vi "Add Noise.vi"(6 "Sampling":T1 {"Fs" format="%#_13g"}, 8 "error in (no error)":errorcluster, 11 "AI []":waveform(dbl)[](array[waveform])) -> (0 "error out":errorcluster, 3 "AI + Noise":waveform(dbl)[](array[waveform]))   [LabVIEW 2019, in "Instrument.Lockin.lvlib" / "Instrument.DAQ.lvclass"]
uses:
  Instrument.DAQ.lvclass
  Typedefs/DAQ.Sampling.Sampling--Cluster.ctl
  <vilib>/measure/maspectr.llb/FFT Power Spectrum and PSD for N Chan.vi
  <vilib>/measure/NI_MABase.lvlib
  <vilib>/measure/NI_MAPro.lvlib
panel:
  out "Waveform Graph":cluster{"f0":dbl, "df":dbl, "magnitude":dbl[]}[](graph)
  in  "Noise Cluster":T2={"1/f vs. Uniform "=1.0, "60Hz Amplitude"=0.005, "Gauss/Unif %"=0.5, "Noise Amp"=0.005}
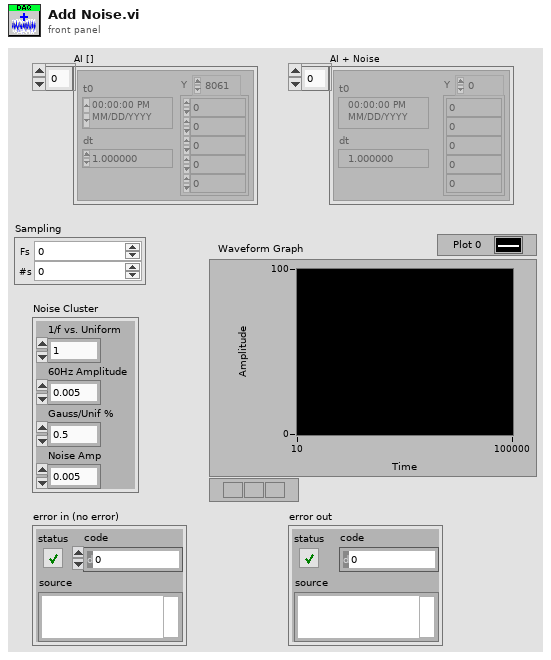
[diagram p1: front panel]
types:
  T1 = typedef "Instrument.Lockin.lvlib/Instrument.DAQ.lvclass/DAQ.Sampling.Sampling--Cluster.ctl" = cluster{"Fs":dbl, "#s":i32}
  T2 = cluster{"1/f vs. Uniform ":dbl, "60Hz Amplitude":dbl, "Gauss/Unif %":dbl, "Noise Amp":dbl}
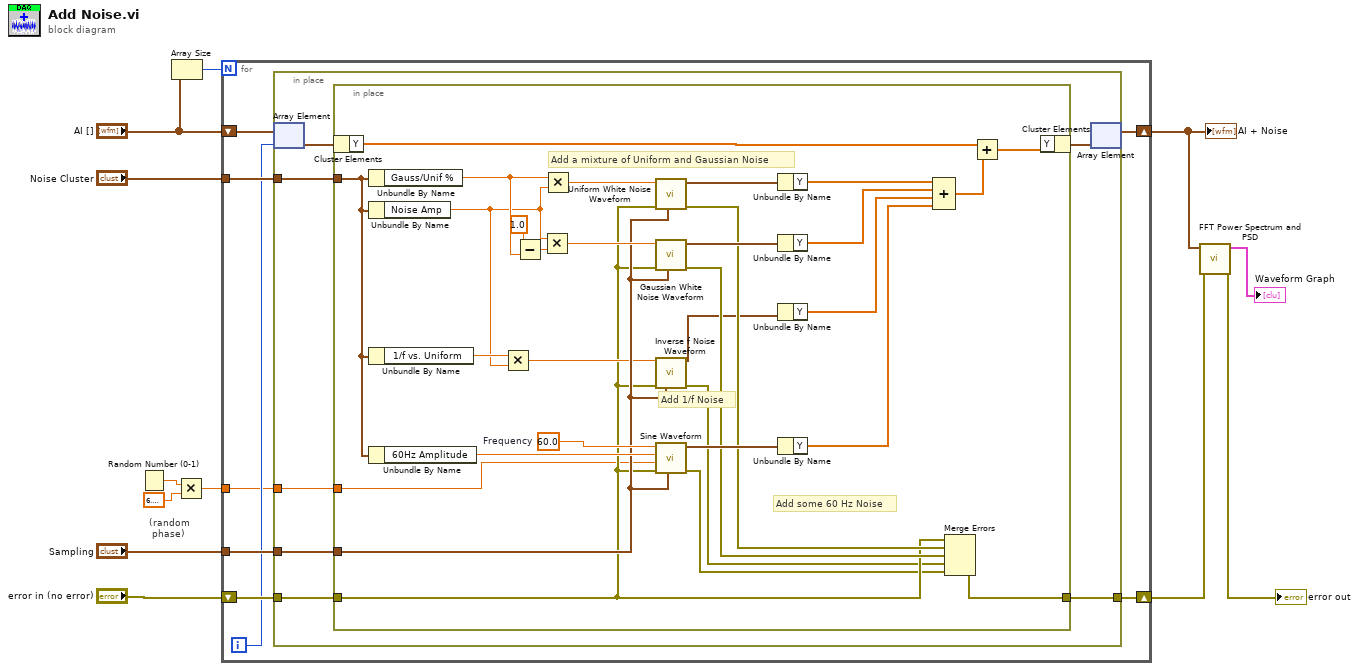
[diagram p0: block diagram]
diagram:
  # "(random\n phase)"
  n1 = Random Number (0-1)() -> (number: 0 to 1=w1:dbl)
  n2 = Array Size(array="AI []") -> (size(s)=w5:i32)
  n3 = Multiply(x=w1, y=6.283185307179586) -> (x*y=w2:dbl)
  n4 = for {
    N: w5 -> [_]
    tunnel: "Noise Cluster" -> [w20]
    tunnel: "Sampling" -> [w19]
    shift-right: [w17] -> w9
    shift-left: "error in (no error)" -> [w18]
    shift-right: [w14] -> w6
    shift-left: "AI []" -> [w16]
    tunnel: w2 -> [w13]
    i -> [w15]
    n5 = in-place {
      in-place-border: w20 -> [w27]
      in-place-border: w19 -> [w26]
      in-place-border: w18 -> [w25]
      in-place-border: [w24] -> w17
      in-place-border: w13 -> [w21]
      n6 = in-place-array #1(w16, w15) -> (w23:waveform(dbl))
      n7 = in-place {
        in-place-border: w27 -> [w57]
        in-place-border: w26 -> [w39]
        in-place-border: w25 -> [w35]
        in-place-border: [w34] -> w24
        in-place-border: w21 -> [w28]
        w43 = 60.0  # Frequency
        # "Add 1/f Noise"
        # "Add some 60 Hz Noise"
        # "Add a mixture of Uniform and Gaussian Noise"
        n8 = in-place-cluster #2(w23) -> ("Y"=w32:dbl[])
        n9 = Unbundle By Name(w57) -> ("Gauss/Unif %"=w48:dbl)
        n10 = Unbundle By Name(w57) -> ("Noise Amp"=w40:dbl)
        n11 = Unbundle By Name(w57) -> ("1/f vs. Uniform"=w47:dbl)
        n12 = Unbundle By Name(w57) -> ("60Hz Amplitude"=w46:dbl)
        n13 = Multiply(x=w47, y=w40) -> (x*y=w38:dbl)
        n14 = Subtract(x=1.0, y=w48) -> (x-y=w54:dbl)
        n15 = Multiply(x=w40, y=w54) -> (x*y=w45:dbl)
        n16 = Multiply(x=w48, y=w40) -> (x*y=w44:dbl)
        n17 = call <vilib>:"Uniform White Noise Waveform.vi"("sampling info"=w39, "error in (no error)"=w35, "amplitude"=w44) -> ("error out"=w41:errorcluster, "signal out"=w55:waveform(dbl))  [unwired: 7 in]
        n18 = call <vilib>:"Gaussian White Noise Waveform.vi"("sampling info"=w39, "error in (no error)"=w35, "standard deviation"=w45) -> ("error out"=w42:errorcluster, "signal out"=w56:waveform(dbl))  [unwired: 7 in]
        n19 = call <vilib>:"Inverse f Noise Waveform.vi"("noise density"=w38, "error in (no error)"=w35, "sampling info"=w39) -> ("signal out"=w37:waveform(dbl), "error out"=w29:errorcluster)  [unwired: 8 in, 3 out]
        n20 = call <vilib>:"Sine Waveform.vi"("sampling info"=w39, "error in (no error)"=w35, "phase"=w28, "amplitude"=w46, "frequency"=w43) -> ("error out"=w30:errorcluster, "signal out"=w52:waveform(dbl))  [unwired: 5 in]
        n21 = Unbundle By Name(w55) -> ("Y"=w51:dbl[])
        n22 = Unbundle By Name(w56) -> ("Y"=w49:dbl[])
        n23 = Unbundle By Name(w37) -> ("Y"=w36:dbl[])
        n24 = Unbundle By Name(w52) -> ("Y"=w50:dbl[])
        n25 = Compound Arithmetic op=ADD(w51, w49, w36, w50) -> (w33:dbl[])
        n26 = Merge Errors(w35, w41, w42, w29, w30) -> (w34:errorcluster)
        n27 = Add(x=w32, y=w33) -> (x+y=w31:dbl[])
        n28 = in-place-cluster #2("Y"=w31) -> (w22:waveform(dbl))
      }
      n29 = in-place-array #1(w22) -> (w14:waveform(dbl)[])  [unwired: 1 out]
    }
  }
  "AI + Noise" <- w6
  n30 = call-poly <vilib>:"FFT Power Spectrum and PSD.vi"("error in (no error)"=w9, "time signals"=w6) -> ("error out"=→"error out":errorcluster, "Power Spectrum / PSD"=→"Waveform Graph":cluster{"f0":dbl, "df":dbl, "magnitude":dbl[]}[])  [unwired: 6 in, 2 out]
